vi "usb reinitialize.vi"(8 "error in (no error)":errorcluster, 11 "foundcards":i32) -> (0 "error out":errorcluster, 2 "function return":i32, 3 "foundcards out":i32)   [LabVIEW 2015, in "SCANalone4x64.lvlib"]
doc: "__declspec(dllimport) long __stdcall usb_reinitialize(long *foundcards);"
uses:
  <userlib>/SCANalone4x64/SCANalone4x64.lvlib
  <userlib>/SCANalone4x64/SCANalone4x64.dll
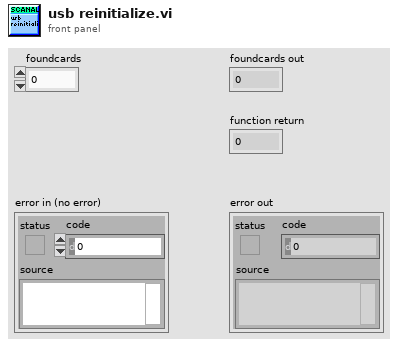
[diagram p1: front panel]
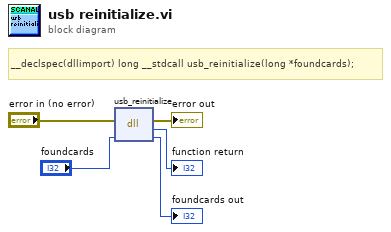
[diagram p0: block diagram]
diagram:
  # "__declspec(dllimport) long __stdcall usb_reinitialize(long *foundcards);"
  n1 = dll-call lib="C:/Program Files/National Instruments/LabVIEW 2015/user.lib/SCANalone4x64/SCANalone4x64.*" fn="usb_reinitialize"(error in="error in (no error)", "foundcards"="foundcards") -> (error out=→"error out":errorcluster, →"function return":i32, "foundcards"=→"foundcards out":i32)  [unwired: 2 in, 1 out]
